vi "Caps_GUI2.vi"(10 "stop 2":refnum<vi>, 11 "GUI_cluster":T1={"Sub Panel"=refnum, "GUIdevice"="Bella_LP_Mode", "CtlRef"=refnum, "user event out"=refnum}) -> ()   [LabVIEW 2013]
uses:
  GUI_Template/GUI_master/tcp_new_data_event.ctl
  GUI_Template/GUI_master/tcp new data cluster.ctl
  Controls/GUI_cluster.ctl
  Controls/eventtypdef.ctl
panel:
  in  "dischargeTime2::8":dbl caption="DisTime2 (ns)" min=-5000.0 max=5000.0
  in  "flow::4":dbl=75.28 caption="flow" min=0.0 max=0.0
  in  "flow::5":dbl=74.96 caption="flow" min=0.0 max=0.0
  out "GUIdevice 8":string="StagingInterlock"
  out "GUIdevice 7":string="StagingInterlock"
  in  "installed.cap2::7":bool caption="CAP2 installed"
  in  "installed.cap1::7":bool caption="CAP1 installed"
  out "read voltage 2":dbl=-0.022297334844 caption="read \nvoltage" min=0.0 max=0.0
  out "read voltage":dbl=0.036783739484999994 caption="read \nvoltage" min=0.0 max=0.0
  out "GUIdevice 6":string="StagingAnalysisSlow"
  out "GUIdevice 5":string="StagingLowPressure2"
  out "GUIdevice 4":string="StagingLowPressure1"
  out "GUIdevice 3":string="StagingNISwitch"
  out "GUIdevice 2":string="StagingDischargePower"
  in  "dischargeTime::8":dbl caption="DisTime1 (ns)" min=-5000.0 max=5000.0
  out "pressureCap1::6":dbl=74.657900037871 caption="pressure read" min=0.0 max=10.0
  out "pressureCap2::6":dbl=77.24427975638 caption="pressure read" min=0.0 max=10.0
  in  "pressure::5":dbl=74.96 caption="pressure" min=0.0 max=300.0
  in  "pressure::4":dbl=75.28 caption="pressure" min=0.0 max=300.0
  in  "discharge2::3":bool caption="Trigger"
  in  "discharge1::3":bool caption="Trigger"
  out "AI_mean.Channel 3::2":dbl=0.012277955671 caption="read \nvoltage" min=0.0 max=0.0
  in  "voltage.hv 2::1":dbl=0.040871 caption="set \nvoltage" min=0.0 max=30.0
  out "AI_mean.Channel 0::2":dbl=-0.007397741276 caption="read \nvoltage" min=0.0 max=0.0
  in  "voltage.hv 1::1":dbl=-0.024775 caption="set \nvoltage" min=0.0 max=30.0
  out "tcp data event":T2
  out "GUIdevice 1":string="StagingDischargeHV"
  in  "stop":bool=TRUE
  # "CAP2"
  # "CAP1"
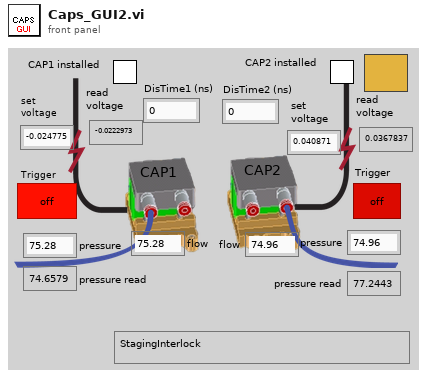
[diagram p1: front panel]
types:
  T1 = typedef "GUI_cluster.ctl" = cluster{"Sub Panel":refnum<vi>, "GUIdevice":string, "CtlRef":refnum<vi>, "user event out":refnum<user-event>}
  T2 = typedef "tcp_new_data_event.ctl" = refnum<user-event>
  T3 = typedef "eventtypdef.ctl" = cluster{"label":string, "Sub Panel":refnum<vi>, "CtlRef":refnum<vi>, "This VI":refnum<vi>}
  T4 = typedef "tcp new data cluster.ctl" = cluster{"EventEnum":enum16{"new data", "connection status update"}, "Device name":string}
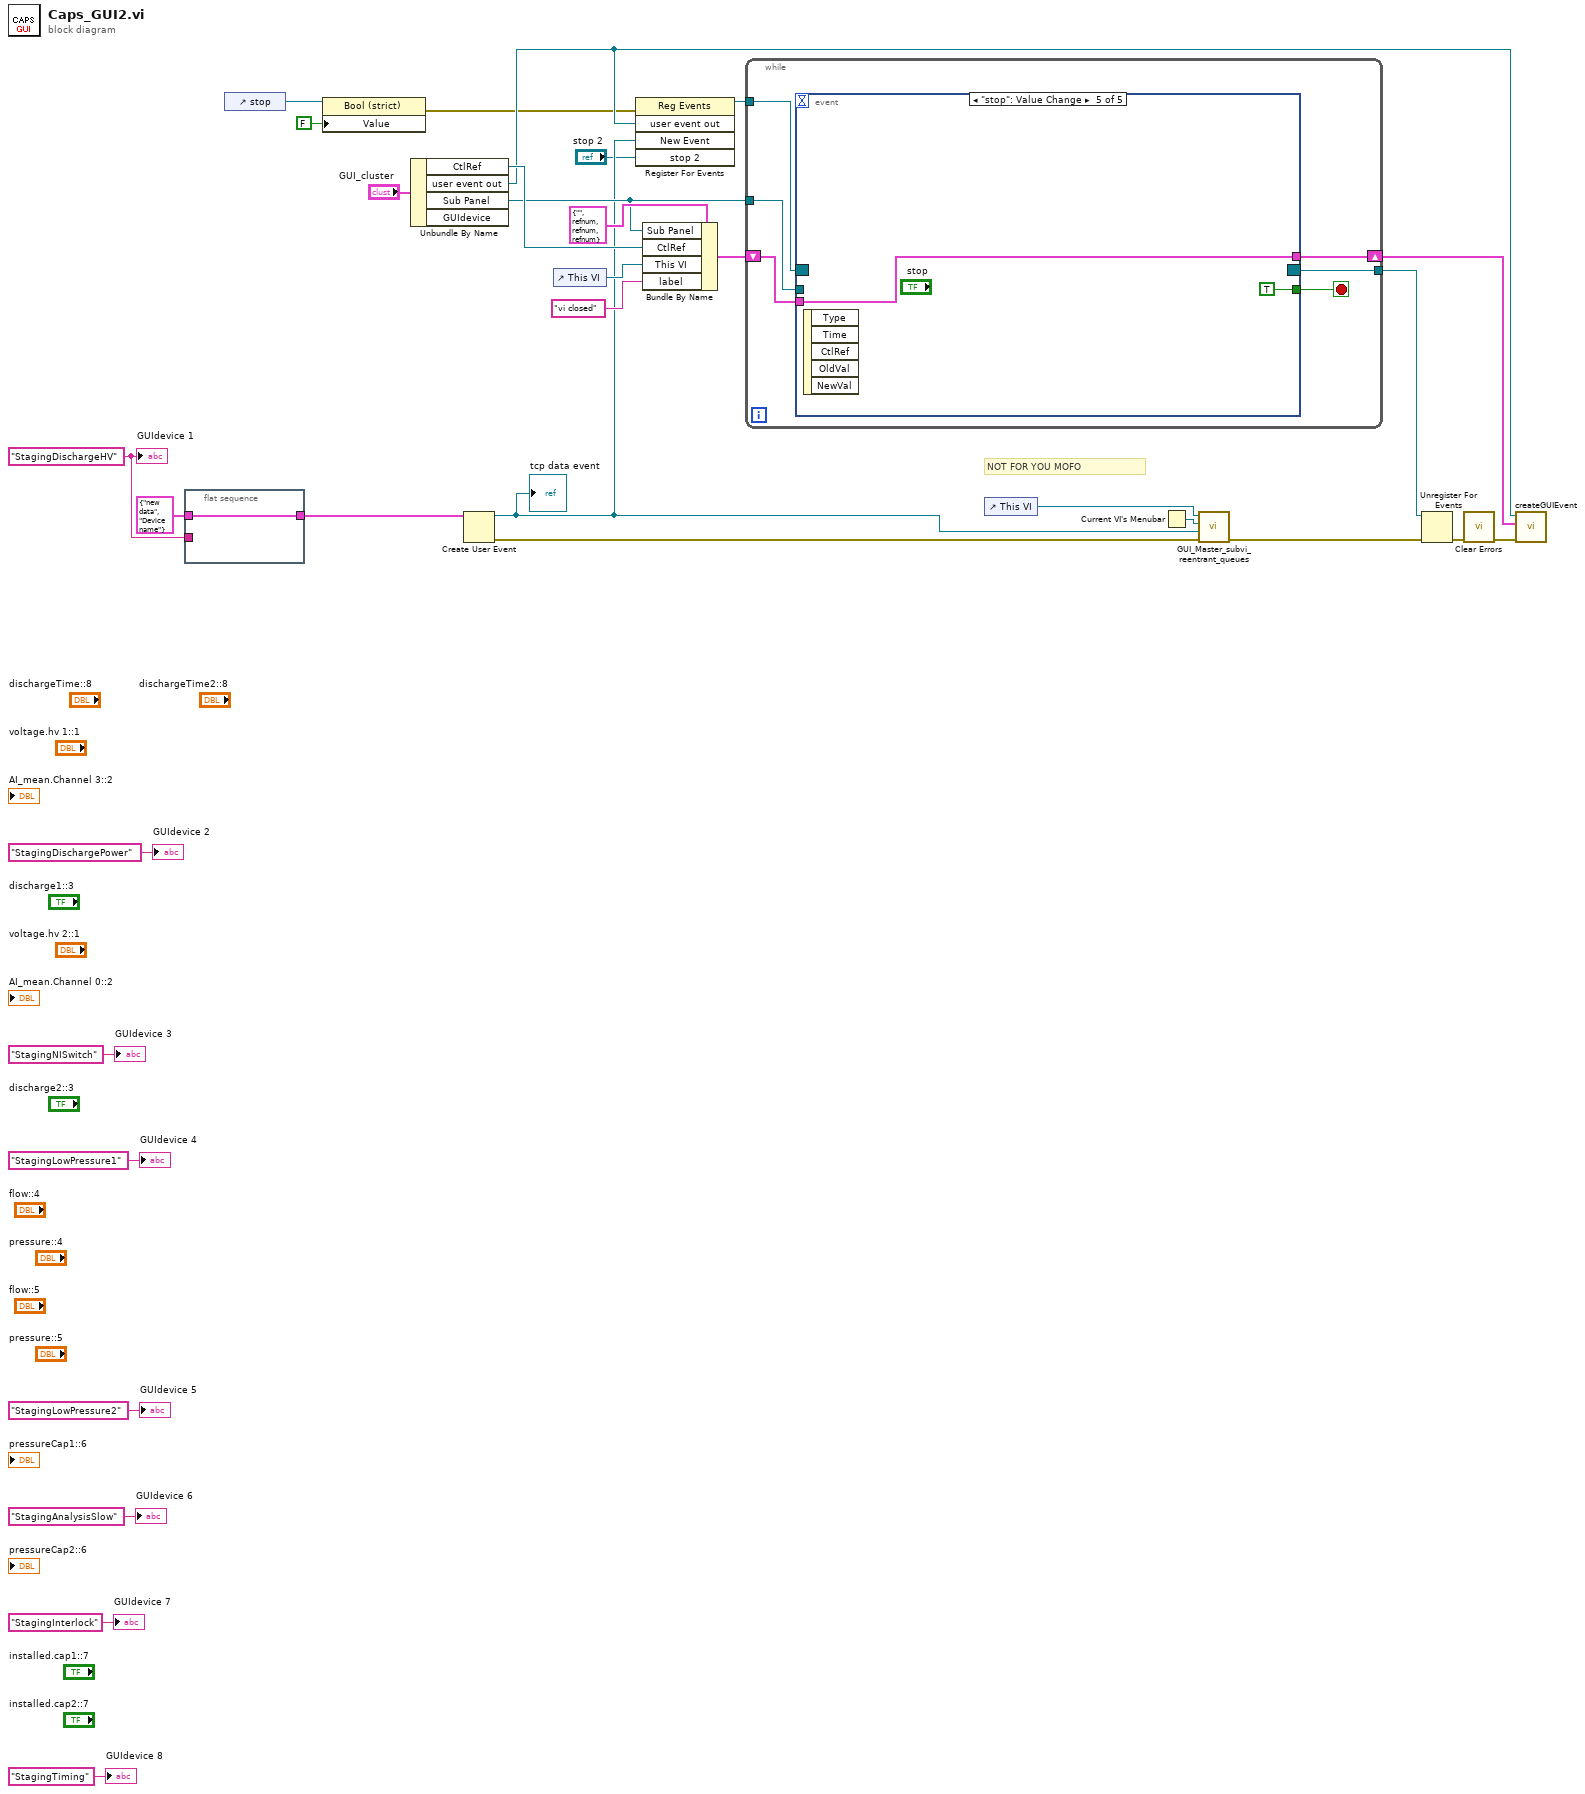
[diagram p0: block diagram]
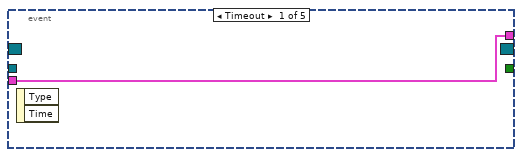
[diagram p2: hidden frame]
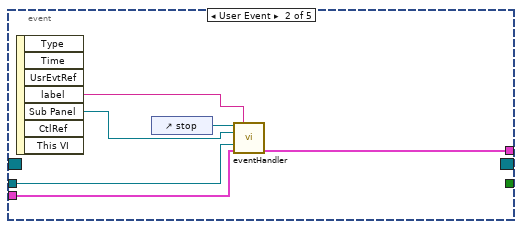
[diagram p3: hidden frame]
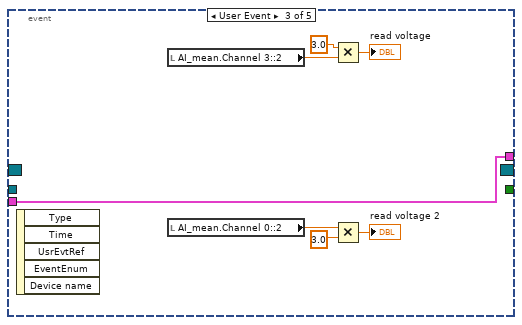
[diagram p4: hidden frame]
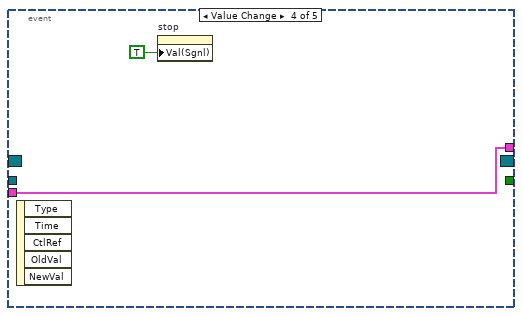
[diagram p5: hidden frame]
diagram:
  w23 = "StagingDischargeHV" ("GUIdevice 23")
  # "NOT FOR YOU MOFO"
  n1 = flat-sequence {
    tunnel: T4 {"EventEnum"=enum."new data", "Device name"="Device name"} ("New Event") -> [w33]
    tunnel: [w33] -> w26
    tunnel: w23 -> [_]
    frame #0 {
    }
  }
  n2 = control-ref of="stop"() -> (w6:refnum<vi>)
  n3 = property class="Bool (strict)"(reference=w6, "Value"=FALSE) -> (error out=w9:errorcluster)  [unwired: 1 in, 1 out]
  n4 = Unbundle By Name("GUI_cluster") -> ("CtlRef"=w25:refnum<vi>, "user event out"=w13:refnum<user-event>, "Sub Panel"=w15:refnum<vi>)  [unwired: 1 out]
  n5 = Create User Event(user event datatype=w26) -> (user event=w11:refnum<user-event>, error out=w30:errorcluster)  [unwired: 1 in]
  "tcp data event" <- w11
  n6 = control-ref of="This VI"() -> (w24:refnum<vi>)
  n7 = register-events(error in=w9, w13, w11, "stop 2") -> (reference out=w17:refnum<event-registration>)  [unwired: 1 in, 1 out]
  n8 = Bundle By Name(cluster=T3 {"label"="", "Sub Panel"=refnum, "CtlRef"=refnum, "This VI"=refnum} ("event data"), "Sub Panel"=w15, "CtlRef"=w25, "This VI"=w24, "label"="vi closed") -> (w14:T3)
  n9 = while {
    tunnel: w17 -> [w39]
    tunnel: w15 -> [w37]
    shift-right: [w35] -> w12
    shift-left: w14 -> [w36]
    tunnel: [w34] -> w4
    stop <- w38 stop-if-true
    n10 = event shown="[4] \"stop\": Value Change" {
      selector: w39 -> [_ _ _ _ _]
      dyn-events: [_ _ _ _ _] -> w34
      timeout: _ -> [_ _ _ _ _]
      tunnel: [_ _ _ _ TRUE ("stop")] -> w38
      tunnel: w37 -> [_ w43 _ _ _]
      tunnel: w36 -> [w40 w42 w47 w55 w57]
      tunnel: [w40 w41 w47 w55 w57] -> w35
      event Timeout {
        n11 = event-data() -> ()  [unwired: 1 in, 2 out]
      }
      event User Event {
        n12 = event-data() -> ("label"=w45:string, "Sub Panel"=w44:refnum<vi>)  [unwired: 1 in, 5 out]
        n13 = control-ref of="stop"() -> (w46:refnum<vi>)
        n14 = call "eventHandler.vi"("Boolean in"=w46, "label"=w45, "Sub Panel 2"=w44, "Sub Panel"=w43, "event data in"=w42) -> ("event data out"=w41:T3)  [unwired: 10 in]
      }
      event User Event {
        n15 = event-data() -> ()  [unwired: 1 in, 5 out]
        n16 = local read "AI_mean.Channel 3::2"() -> (w53:dbl)
        n17 = local read "AI_mean.Channel 0::2"() -> (w50:dbl)
        n18 = Multiply(x=3.0, y=w53) -> (x*y=→"read voltage":dbl)
        n19 = Multiply(x=w50, y=3.0 ("x")) -> (x*y=→"read voltage 2":dbl)
      }
      event Value Change {
        n20 = event-data() -> ()  [unwired: 1 in, 5 out]
        n21 = property on="stop" class="Bool (strict)"("Val(Sgnl)"=TRUE ("Value (Signaling)")) -> ()  [unwired: 2 in, 2 out]
      }
      event "stop": Value Change {
        n22 = event-data() -> ()  [unwired: 1 in, 5 out]
      }
    }
  }
  n23 = control-ref of="This VI"() -> (w32:refnum<vi>)
  n24 = Current VI's Menubar() -> (w31:refnum<k9>)
  n25 = call "GUI_Master_subvi_reentrant_queues.vi"("error in (no error)"=w30, "tcp data event"=w11, "Caller menu reference"=w31, "Caller VI ref"=w32) -> ("error out"=w2:errorcluster)  [unwired: 7 in]
  n26 = Unregister For Events(event registration refnum=w4, error in=w2) -> (error out=w3:errorcluster)
  n27 = call <vilib>:"Clear Errors.vi"("error in (no error)"=w3) -> ("error out"=w1:errorcluster)  [unwired: 6 in]
  n28 = call "createGUIEvent.vi"("error in (no error)"=w1, "event data"=w12, "User Event in"=w13) -> ()  [unwired: 8 in, 1 out]
  "GUIdevice 1" <- w23
  "GUIdevice 2" <- "StagingDischargePower" ("GUIdevice 23")
  "GUIdevice 3" <- "StagingNISwitch" ("GUIdevice 8")
  "GUIdevice 4" <- "StagingLowPressure1" ("GUIdevice 2")
  "GUIdevice 5" <- "StagingLowPressure2" ("GUIdevice 2")
  "GUIdevice 6" <- "StagingAnalysisSlow" ("GUIdevice 1")
  "GUIdevice 7" <- "StagingInterlock" ("GUIdevice 7")
  "GUIdevice 8" <- "StagingTiming" ("GUIdevice 7")
